vi "HP 3325B - Set Phase (SubVI).vi"(6 "write_delay (ms)":u32=20, 7 "GPIB Address":string="11", 8 "error_in":errorcluster, 9 "write?":bool=TRUE, 11 "phase (deg)":ext format="%.3f") -> (0 "error out":errorcluster, 3 "command string":string)   [LabVIEW 2018]
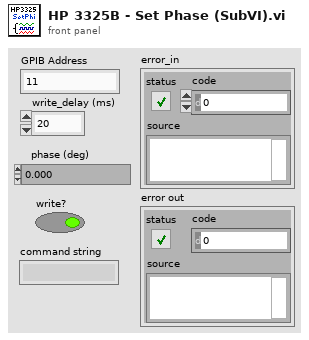
[diagram p1: front panel]
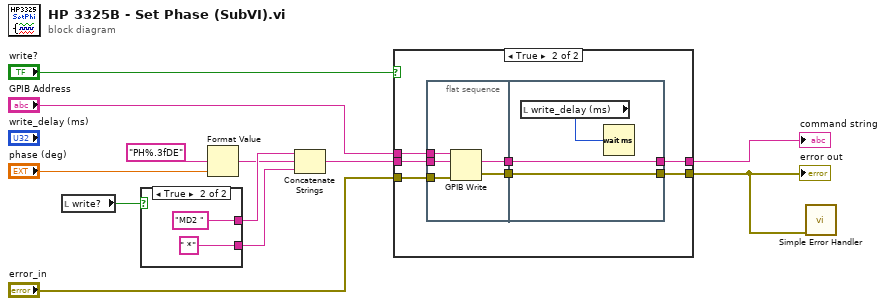
[diagram p0: block diagram]
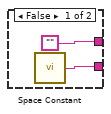
[diagram p2: hidden frame]
diagram:
  n1 = local read "write?"() -> (w1:bool)
  n2 = case shown="True" w1 {
    tunnel: [w14 " *"] -> w5
    tunnel: ["" "MD2 " ("string (\"\")")] -> w7
    frame False {
      n3 = call <vilib>:"Space Constant.vi"() -> ("String"=w14:string)
    }
    frame True {
    }
  }
  n4 = Format Value(format string="PH%.3fDE", value (0)="phase (deg)") -> (output string=w6:string)  [unwired: 1 in]
  n5 = Concatenate Strings(w7, w6, w5) -> (w4:string)
  n6 = case shown="True" "write?" {
    tunnel: [w18 w24] -> w12
    tunnel: w4 -> [w17 w23]
    tunnel: "error_in" -> [w18 w22]
    tunnel: "GPIB Address" -> [_ w21]
    tunnel: [w17 w19] -> w8
    frame False {
    }
    frame True {
      n7 = flat-sequence {
        tunnel: w21 -> [w29]
        tunnel: w23 -> [w26]
        tunnel: w22 -> [w27]
        tunnel: [w28] -> w25
        tunnel: [w26] -> w20
        tunnel: [w32] -> w24
        tunnel: w25 -> [w32]
        tunnel: w20 -> [w30]
        tunnel: [w30] -> w19
        frame #0 {
          n8 = GPIB Write(0:w29, 1:w26, 3:w27) -> (6:w28:errorcluster)  [unwired: 2 in, 1 out]
        }
        frame #1 {
          n9 = local read "write_delay (ms)"() -> (w31:u32)
          n10 = Wait (ms)(milliseconds to wait=w31) -> ()  [unwired: 1 out]
        }
      }
    }
  }
  "error out" <- w12
  "command string" <- w8
  n11 = call <vilib>:"Simple Error Handler.vi"("error in (no error)"=w12) -> ()  [unwired: 4 in, 5 out]
